vi "kuvaitech_2.vi"() -> ()   [LabVIEW 2021]
uses:
  <vilib>/LabVIEW Interface for Arduino/Type Defs/Board Type.ctl
  <vilib>/LabVIEW Interface for Arduino/Type Defs/Pin Mode.ctl
  <vilib>/LabVIEW Interface for Arduino/LabVIEW Interface for Arduino.lvlib
panel:
  in  "Boolean":bool
  in  "Digital I/O Pin":u8
  in  "stop":bool
  in  "Board Type (Uno)":T1
  in  "VISA resource":refnum<visa-resource-name>
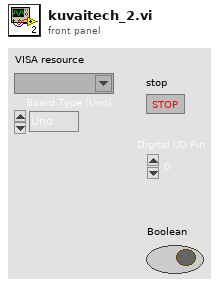
[diagram p1: front panel]
types:
  T1 = typedef "LabVIEW Interface for Arduino.lvlib/Board Type.ctl" = enum16{"Uno", "Dimuelanove w/Atmega 328", "Mega 2560"}
  T2 = typedef "LabVIEW Interface for Arduino.lvlib/Pin Mode.ctl" = enum8{"Input", "Output"}
  T3 = typedef "LabVIEW Interface for Arduino.lvlib/Arduino Resource.ctl" = cluster{"VISA resource":refnum<visa-resource-name>, "Board Type":T1, "Connection Type":enum8{"USB / Serial"}, "Bytes Per Packet (15)":u8}
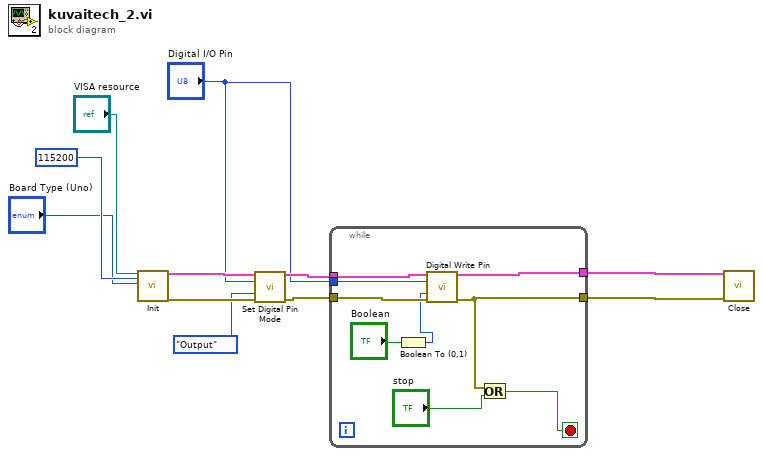
[diagram p0: block diagram]
diagram:
  n1 = call <vilib>:"Init.vi"("VISA resource"="VISA resource", "Baud Rate (115200)"=u32 115200, "Board Type (Uno)"="Board Type (Uno)") -> ("Arduino Resource"=w8:T3, "error out"=w5:errorcluster)  [unwired: 15 in]
  n2 = call <vilib>:"Set Digital Pin Mode.vi"("Arduino Resource"=w8, "Digital I/O Pin"="Digital I/O Pin", "Pin Mode (Input)"=Pin_Mode."Output", "error in"=w5) -> ("Arduino Resource"=w7:T3, "error out"=w4:errorcluster)  [unwired: 10 in]
  n3 = while {
    tunnel: w7 -> [w20]
    tunnel: [w19] -> w6
    tunnel: w4 -> [w18]
    tunnel: [w15] -> w3
    tunnel: "Digital I/O Pin" -> [w12]
    stop <- w16 stop-if-true
    n4 = Boolean To (0,1)(Boolean="Boolean") -> (0, 1=w14:i16)
    n5 = call <vilib>:"Digital Write Pin.vi"("Arduino Resource"=w20, "Digital I/O Pin (0)"=w12, "Value (0)"=w14, "error in"=w18) -> ("Arduino Resource"=w19:T3, "error out"=w15:errorcluster)  [unwired: 10 in]
    n6 = Or(x=w15, y="stop") -> (x .or. y?=w16:bool)
  }
  n7 = call <vilib>:"Close.vi"("Arduino Resource"=w6, "error in"=w3) -> ()  [unwired: 13 in, 1 out]
